vi "ExSubBuildColor.vi"(1 "Count":u32=256 min=2 step=1, 2 "End Color":u32, 3 "Start Color":u32) -> (0 "Array":i32[](array[numeric]))   [LabVIEW 2010]
uses:
  <vilib>/Platform/NI_3dgraph.lvlib
panel:
  # "ExSubBuildColor: builds up pseudo color table"
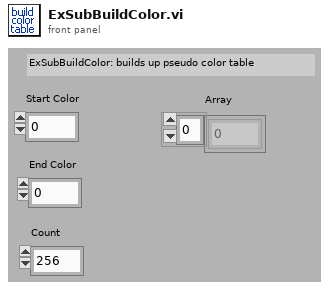
[diagram p1: front panel]
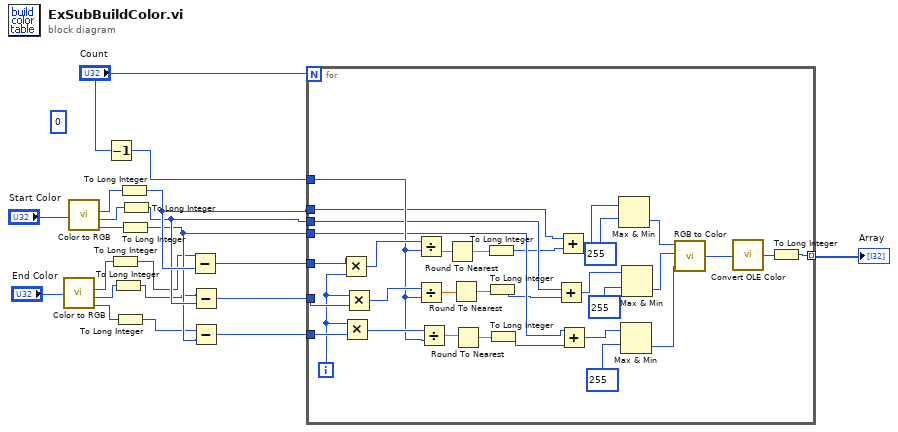
[diagram p0: block diagram]
diagram:
  (unwired) 0
  n1 = call <vilib>:"Color to RGB.vi"("Color"="End Color") -> ("R"=w6:u8, "G"=w4:u8, "B"=w2:u8)  [unwired: 1 out]
  n2 = call <vilib>:"Color to RGB.vi"("Color"="Start Color") -> ("R"=w12:u8, "G"=w10:u8, "B"=w8:u8)  [unwired: 1 out]
  n3 = Decrement(x="Count") -> (x-1=w15:u32)
  n4 = To Long Integer(number=w6) -> (32bit integer=w5:i32)
  n5 = To Long Integer(number=w4) -> (32bit integer=w3:i32)
  n6 = To Long Integer(number=w2) -> (32bit integer=w1:i32)
  n7 = To Long Integer(number=w12) -> (32bit integer=w11:i32)
  n8 = To Long Integer(number=w8) -> (32bit integer=w7:i32)
  n9 = To Long Integer(number=w10) -> (32bit integer=w9:i32)
  n10 = Subtract(x=w5, y=w11) -> (x-y=w18:i32)
  n11 = Subtract(x=w3, y=w9) -> (x-y=w17:i32)
  n12 = Subtract(x=w1, y=w7) -> (x-y=w16:i32)
  n13 = for {
    N: "Count" -> [_]
    tunnel: w11 -> [w44]
    tunnel: w9 -> [w43]
    tunnel: w7 -> [w42]
    tunnel: w18 -> [w50]
    tunnel: w17 -> [w51]
    tunnel: w16 -> [w52]
    tunnel: w15 -> [w45]
    tunnel: [w22] -> w13 mode=indexing
    i -> [w49]
    n14 = Multiply(x=w50, y=w49) -> (x*y=w46:i32)
    n15 = Multiply(x=w49, y=w52) -> (x*y=w48:i32)
    n16 = Multiply(x=w49, y=w51) -> (x*y=w47:i32)
    n17 = Divide(x=w46, y=w45) -> (x/y=w41:dbl)
    n18 = Divide(x=w47, y=w45) -> (x/y=w38:dbl)
    n19 = Divide(x=w48, y=w45) -> (x/y=w35:dbl)
    n20 = Round To Nearest(number=w41) -> (nearest integer value=w40:dbl)
    n21 = Round To Nearest(number=w38) -> (nearest integer value=w37:dbl)
    n22 = Round To Nearest(number=w35) -> (nearest integer value=w34:dbl)
    n23 = To Long Integer(number=w40) -> (32bit integer=w39:i32)
    n24 = To Long Integer(number=w37) -> (32bit integer=w36:i32)
    n25 = To Long Integer(number=w34) -> (32bit integer=w33:i32)
    n26 = Add(x=w43, y=w36) -> (x+y=w27:i32)
    n27 = Add(x=w44, y=w39) -> (x+y=w28:i32)
    n28 = Add(x=w42, y=w33) -> (x+y=w31:i32)
    n29 = Max & Min(x=w28, y=255) -> (min(x,y)=w26:i32)  [unwired: 1 out]
    n30 = Max & Min(x=w31, y=255) -> (min(x,y)=w24:i32)  [unwired: 1 out]
    n31 = Max & Min(x=w27, y=255) -> (min(x,y)=w25:i32)  [unwired: 1 out]
    n32 = call <vilib>:"RGB to Color.vi"("B"=w24, "G"=w25, "R"=w26) -> ("Color"=w23:u32)
    n33 = call <vilib>:"Convert OLE Color.vi"("color in"=w23) -> ("color out"=w21:u32)
    n34 = To Long Integer(number=w21) -> (32bit integer=w22:i32)
  }
  "Array" <- w13
